vi "Read.vi"(8 "error in (no error)":errorcluster, 11 "Maxcon Encoder Simulator in":refnum<class "Maxon Encoder Simulator.lvclass">) -> (0 "error out":errorcluster, 1 "Velocity (rad/Sec)":dbl, 2 "Angular Position (rad)":dbl, 3 "Maxcon Encoder Simulator out":refnum<class "Maxon Encoder Simulator.lvclass">)   [LabVIEW 2019, in "Maxon Encoder Simulator.lvclass"]
doc: "Reads the encoder position."
uses:
  Maxon Encoder Simulator.lvclass
  <resource>/objmgr/LVODE.rc
  <vilib>/robotics/Simulator/Robot Factory/Motor/ODESimulator_Motor.lvclass
  <vilib>/Analysis/NI_AAL_Angle.lvlib
  <vilib>/Analysis/coordinate.llb/Wrap Angle (scalar).vi
  <vilib>/Analysis/coordinate.llb/Angle Range (Degree).ctl
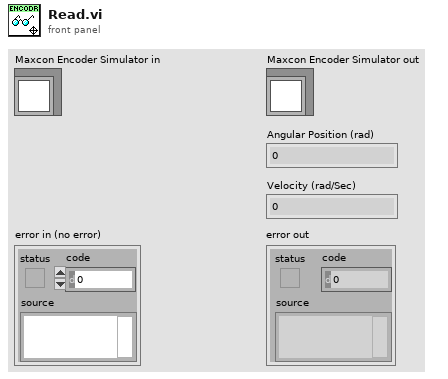
[diagram p1: front panel]
types:
  T1 = typedef "NI_AAL_Angle.lvlib/Angle Range (Degree).ctl" = u16
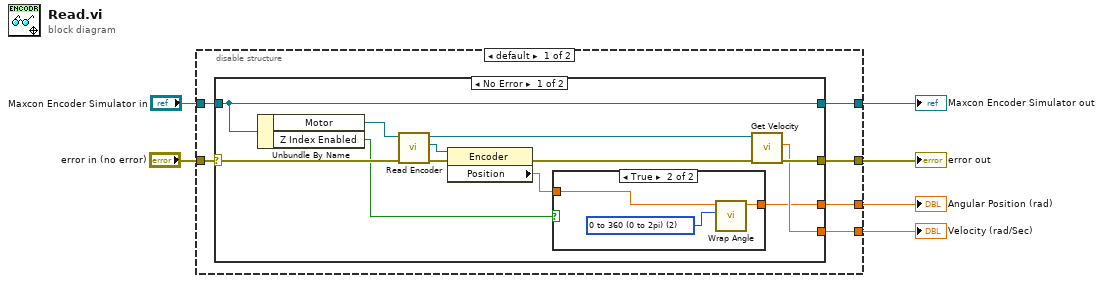
[diagram p0: block diagram]
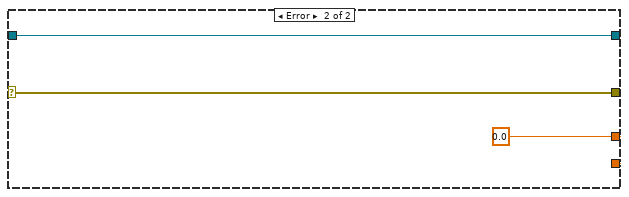
[diagram p3: hidden frame]
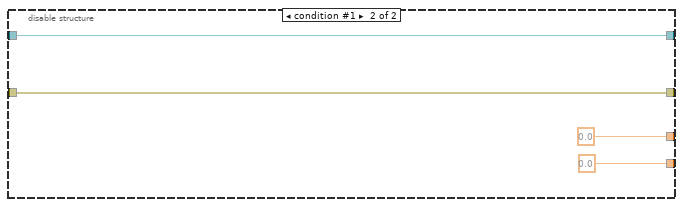
[diagram p4: hidden frame]
diagram:
  n1 = disable-structure shown="default" {
    disable-tunnel: "error in (no error)" -> [w12 w35]
    disable-tunnel: [w11 w35] -> w4
    disable-tunnel: "Maxcon Encoder Simulator in" -> [w10 w34]
    disable-tunnel: [w9 w34] -> w5
    disable-tunnel: [w8 0.0 ("Distance (cm)")] -> w3
    disable-tunnel: [w7 0.0 ("Distance")] -> w2
    frame condition #0 (active) {
      n2 = case shown="No Error" w12 {
        selector: w12 -> [w22 w31]
        tunnel: [w17 w31] -> w11
        tunnel: w10 -> [w24 w30]
        tunnel: [w24 w30] -> w9
        tunnel: [w13 w29] -> w8
        tunnel: [w16 w29] -> w7
        frame No Error {
          n3 = Unbundle By Name(w24) -> ("Motor"=w23:refnum<class "ODESimulator_Motor.lvclass">, "Z Index Enabled"=w15:bool)
          n4 = call <vilib>:"Read Encoder.vi"("error in (no error)"=w22, "ODESimulator_Motor in"=w23) -> ("error out"=w20:errorcluster, "Encoder"=w21:refnum<k20>, "ODESimulator_Motor out"=w19:refnum<class "ODESimulator_Motor.lvclass">)  [unwired: 7 in]
          n5 = property class="Encoder"(reference=w21, error in=w20) -> (error out=w18:errorcluster, "Position"=w14:sgl)  [unwired: 1 out]
          n6 = case shown="True" w15 {
            tunnel: w14 -> [w25 w28]
            tunnel: [w25 w27] -> w13
            frame False {
            }
            frame True {
              w26 = T1 2 items=["none", "-180 to 180 (-pi to pi)", "0 to 360 (0 to 2pi)"] ("angle range")
              n7 = call-poly <vilib>:"Wrap Angle.vi"("angle range"=w26, "angle in"=w28) -> ("angle out"=w27:dbl)  [unwired: 8 in, 1 out]
            }
          }
          n8 = call-dynamic "Get Velocity.vi"("error in (no error)"=w18, "Motor in"=w19) -> ("error out"=w17:errorcluster, "CCW Velocity (rad/s)"=w16:dbl)  [unwired: 7 in, 1 out]
        }
        frame Error {
          w29 = 0.0 ("Distance")
        }
      }
    }
    frame condition #1 {
    }
  }
  "error out" <- w4
  "Angular Position (rad)" <- w3
  "Maxcon Encoder Simulator out" <- w5
  "Velocity (rad/Sec)" <- w2
